vi "Close Modules.vi"(1 "RSI Modules in":T1[](array[typedef]) {"Module Config Data"."Config Block Data Refs"."Data Reference" format="%.0x"; "CDOutput Data"."BD Refs"."Data Reference" format="%.0x"; "CDInput Data"."BD Refs"."Data Reference" format="%.0x"; "VS ref" format="%.0x"}) -> (0 "RSI Modules out":T1[](array[typedef]) {"Module Config Data"."Config Block Data Refs"."Data Reference" format="%.0x"; "CDOutput Data"."BD Refs"."Data Reference" format="%.0x"; "CDInput Data"."BD Refs"."Data Reference" format="%.0x"; "VS ref" format="%.0x"})   [LabVIEW 2016, in "Scan Engine Custom Device.lvlib"]
uses:
  Scan Engine Custom Device.lvlib
  Modules.lvlibp/RSI Module/RSI Module.lvclass
  <vilib>/NI Veristand/Custom Device API/Custom Device Item Ref.ctl
  <vilib>/NI Veristand/Custom Device API/Custom Device API.lvlib
  <vilib>/NI Veristand/Custom Device API/Data Reference.ctl
  <vilib>/NI Veristand/Custom Device API/Block Data Reference.ctl
  Type Defs/Input Data.ctl
  Type Defs/Output Data.ctl
  Modules.lvlibp/RSI Module/Channel Type.ctl
  Modules.lvlibp/RSI Module/Module Models.ctl
  Type Defs/Module Config Data.ctl
  Type Defs/Mixed IO.ctl
  Type Defs/RSI Module Data.ctl
  Type Defs/Open Module IOVs.ctl
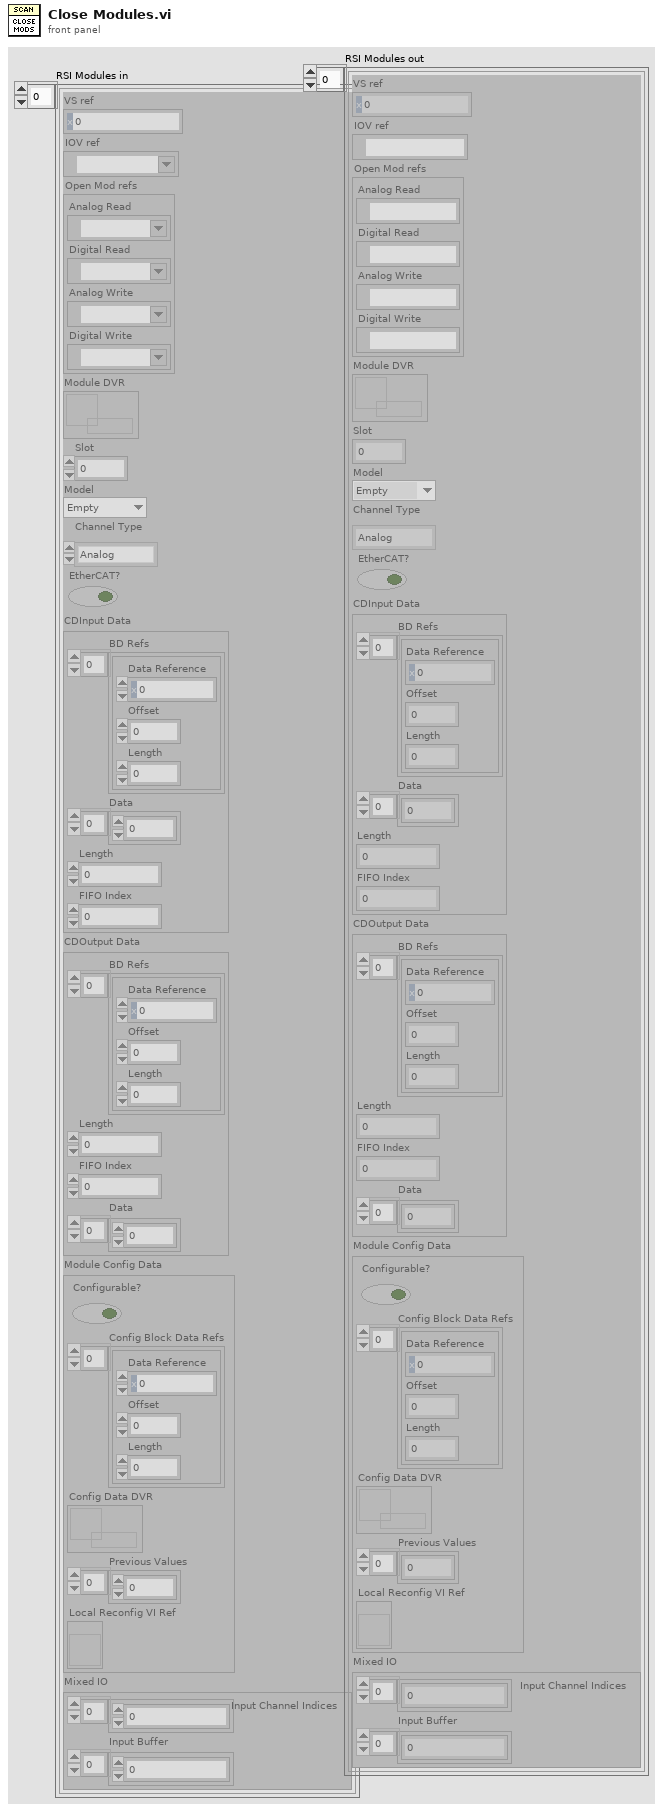
[diagram p1: front panel]
types:
  T1 = typedef "Scan Engine Custom Device.lvlib/RSI Module Data.ctl" = cluster{"VS ref":T2, "IOV ref":refnum<k21>, "Open Mod refs":T3, "Module DVR":refnum<data-value>, "Slot":u32, "Model":T4, "Channel Type":T5, "EtherCAT?":bool, "CDInput Data":T6, "CDOutput Data":T9, "Module Config Data":T10, "Mixed IO":T11}
  T2 = typedef "Custom Device API.lvlib/Custom Device Item Ref.ctl" = u64
  T3 = typedef "Scan Engine Custom Device.lvlib/Open Module IOVs.ctl" = cluster{"Analog Read":refnum<k21>, "Digital Read":refnum<k21>, "Analog Write":refnum<k21>, "Digital Write":refnum<k21>}
  T4 = typedef "Modules.lvlibp/RSI Module.lvclass/Module Models.ctl" = enum16{"Empty", "NI 9201", "NI 9203", "NI 9205", "NI 9206", "NI 9207", "NI 9208", "NI 9211", "NI 9213", "NI 9214", "NI 9215", "NI 9217", "NI 9219", "NI 9221", "NI 9225", "NI 9227", "NI 9229", "NI 9233", "NI 9234", "NI 9235", "NI 9236", "NI 9237", "NI 9239", "NI 9263", "NI 9264", "NI 9265", "NI 9269", "NI 9375", "NI 9401", "NI 9402", "NI 9403", "NI 9411", "NI 9421", "NI 9422", "NI 9423", "NI 9425", "NI 9426", "NI 9435", "NI 9472", "NI 9474", "NI 9475", "NI 9476", "NI 9477", "NI 9478", "NI 9481", "NI 9482", "NI 9485"}
  T5 = typedef "Modules.lvlibp/RSI Module.lvclass/Channel Type.ctl" = enum16{"Analog", "Digital"}
  T6 = typedef "Scan Engine Custom Device.lvlib/Input Data.ctl" = cluster{"BD Refs":T7[], "Data":dbl[], "Length":i32, "FIFO Index":i32}
  T7 = typedef "Custom Device API.lvlib/Block Data Reference.ctl" = cluster{"Data Reference":T8, "Offset":u64, "Length":u64}
  T8 = typedef "Custom Device API.lvlib/Data Reference.ctl" = i32
  T9 = typedef "Scan Engine Custom Device.lvlib/Output Data.ctl" = cluster{"BD Refs":T7[], "Length":i32, "FIFO Index":i32, "Data":dbl[]}
  T10 = typedef "Scan Engine Custom Device.lvlib/Module Config Data.ctl" = cluster{"Configurable?":bool, "Config Block Data Refs":T7[], "Config Data DVR":refnum<data-value>, "Previous Values":dbl[], "Local Reconfig VI Ref":refnum<vi>}
  T11 = typedef "Scan Engine Custom Device.lvlib/Mixed IO.ctl" = cluster{"Input Channel Indices":i32[], "Input Buffer":dbl[]}
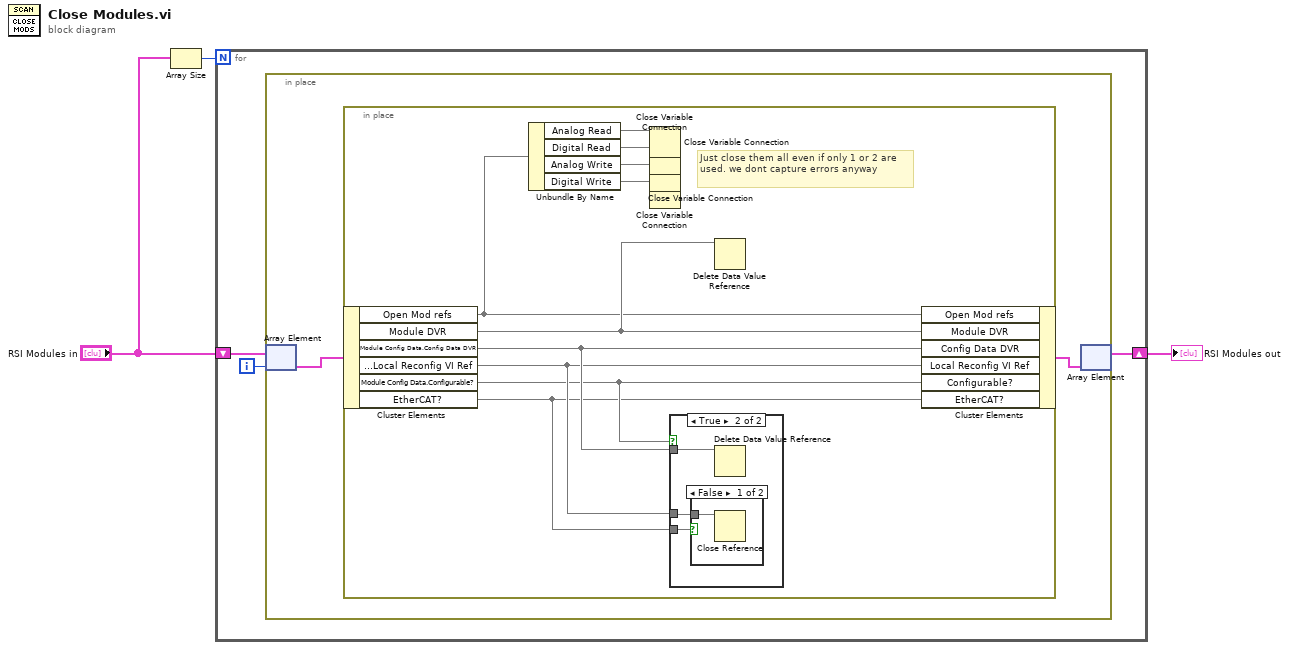
[diagram p0: block diagram]
diagram:
  n1 = Array Size(array="RSI Modules in") -> (size(s)=w1:i32)
  n2 = for {
    N: w1 -> [_]
    shift-right: [w5] -> w3
    shift-left: "RSI Modules in" -> [w6]
    i -> [w4]
    n3 = in-place {
      n4 = in-place-array #1(w6, w4) -> (w8:T1)
      n5 = in-place {
        # "Just close them all even if only 1 or 2 are used. we dont capture errors anyway"
        n6 = in-place-cluster #2(w8) -> ("Open Mod refs"=w13, "Module DVR"=w18, "Module Config Data.Config Data DVR"=w17, "Module Config Data.Local Reconfig VI Ref"=w16, "Module Config Data.Configurable?"=w15, "EtherCAT?"=w14)
        n7 = Unbundle By Name(w13) -> ("Analog Read"=w12, "Digital Read"=w11, "Analog Write"=w10, "Digital Write"=w9)
        n8 = Close Variable Connection(11:w12) -> ()  [unwired: 1 in, 1 out]
        n9 = Close Variable Connection(11:w11) -> ()  [unwired: 1 in, 1 out]
        n10 = Close Variable Connection(11:w10) -> ()  [unwired: 1 in, 1 out]
        n11 = Close Variable Connection(11:w9) -> ()  [unwired: 1 in, 1 out]
        n12 = case shown="True" w15 {
          tunnel: w17 -> [_ w21]
          tunnel: w16 -> [_ w20]
          tunnel: w14 -> [_ w19]
          frame False {
          }
          frame True {
            n13 = case shown="False" w19 {
              tunnel: w20 -> [w22 _]
              frame False {
                n14 = Close Reference(reference=w22) -> ()  [unwired: 1 in, 1 out]
              }
              frame True {
              }
            }
            n15 = Delete Data Value Reference(data value reference=w21) -> ()  [unwired: 1 in, 2 out]
          }
        }
        n16 = Delete Data Value Reference(data value reference=w18) -> ()  [unwired: 1 in, 2 out]
        n17 = in-place-cluster #2("Open Mod refs"=w13, "Module DVR"=w18, "Config Data DVR"=w17, "Local Reconfig VI Ref"=w16, "Configurable?"=w15, "EtherCAT?"=w14) -> (w7:cluster{})
      }
      n18 = in-place-array #1(w7) -> (w5:T1[])  [unwired: 1 out]
    }
  }
  "RSI Modules out" <- w3
